vi "ELVIS III v1.0 Write DO Block Bank B DMA.vi"(8 "error in (no error)":errorcluster, 9 "DO FIFO Clock Divisor":u16, 10 "Bank Data":T1 caption="DO (N Samples) Configuration", 11 "FPGA Reference out":T3) -> (0 "error out":errorcluster)   [LabVIEW 2021]
uses:
  <vilib>/myRIO/Common/Instrument Driver Framework/Utilities/typedefs/Generic FPGA Reference.ctl
  <vilib>/myRIO/Common/Instrument Driver Framework/ELVIS III v1.0/DO Block/typedefs/ELVIS III DO Block Bank Data.ctl
  <vilib>/myRIO/Common/Instrument Driver Framework/ELVIS III v1.0/Resource Manager/typedefs/ELVIS III v1.0 Connector List.ctl
  <vilib>/myRIO/Common/Instrument Driver Framework/ELVIS III v1.0/DO Block/typedefs/ELVIS III DO Block FPGA Reference.ctl
  <vilib>/Utility/error.llb/Error Cluster From Error Code.vi
  <vilib>/rvi/errors/niLvFpgaAdjustHostInterfaceError.vi
  <vilib>/rvi/interface/nirviReadWriteControl/nirviReadWriteControl.xnode
  <vilib>/rvi/interface/nirviMethod/nirviMethod.xnode
  NiFpgaLv.dll
  <vilib>/rvi/interface/Simulation/niFpgaSimulationCallBeginRW.vi
  <vilib>/FPGAPlugInAG/Dynamic/niLvFpga_WriteFifo_Dynamic.vi
  <vilib>/rvi/errors/niLvFpgaMergeErrorWithErrorCode.vi
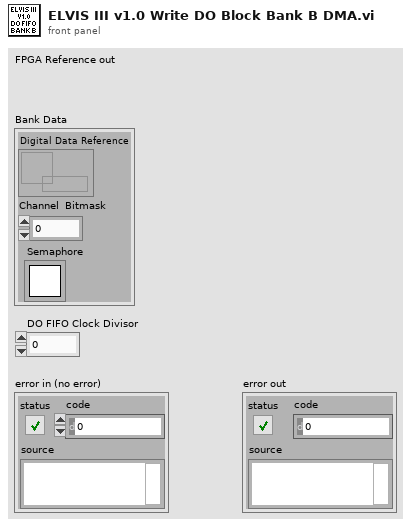
[diagram p1: front panel]
types:
  T1 = typedef "ELVIS III DO Block Bank Data.ctl" = cluster{"Digital Data Reference":refnum<data-value>, "Channel  Bitmask":fxp<+,20,20>, "Semaphore":T2}
  T2 = typedef "Semaphore RefNum" = refnum<k1>
  T3 = typedef "Generic FPGA Reference.ctl" = refnum<k20>
  T4 = typedef "ELVIS III v1.0 Connector List.ctl" = enum32{"None", "ConnectorA", "ConnectorB"}
  T5 = typedef "ELVIS III DO Block FPGA Reference.ctl" = refnum<k20>
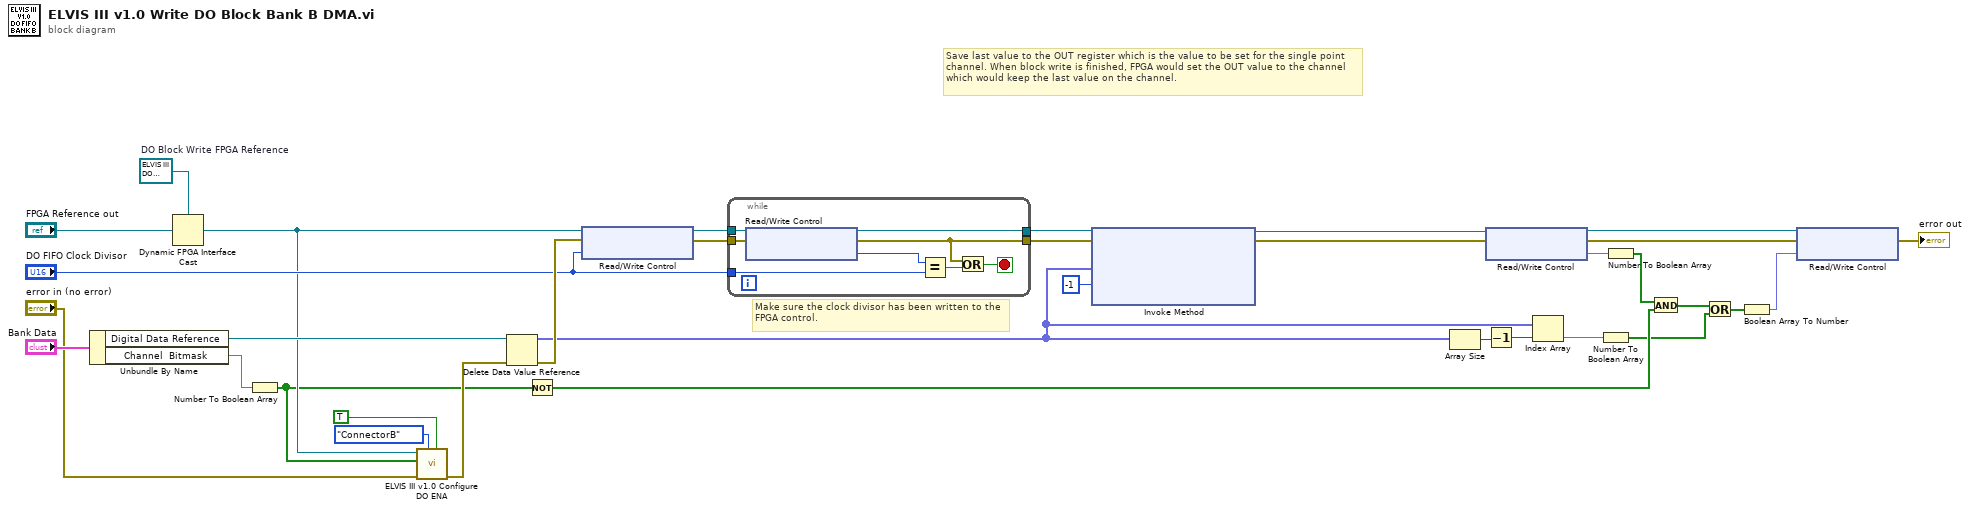
[diagram p0: block diagram]
diagram:
  w34 = T5 refnum  # DO Block Write FPGA Reference
  # "Save last value to the OUT register which is the value to be set for the single point channel. When block write is finished, FPGA would set the OUT value to the channel which would keep the last value on the channel."
  # "Make sure the clock divisor has been written to the FPGA control."
  n1 = Unbundle By Name("Bank Data") -> ("Digital Data Reference"=w14:refnum<data-value>, "Channel  Bitmask"=w13:fxp<+,20,20>)
  n2 = Dynamic FPGA Interface Cast(Session In=w34, Type="FPGA Reference out") -> (Session Out=w4:T5)
  n3 = Number To Boolean Array(number=w13) -> (Boolean array=w3:bool[])
  n4 = call <vilib>:"ELVIS III v1.0 Configure DO ENA.vi"("Apply Bitmask?"=TRUE, "Connector List"=ELVIS_III_v1.0_Connector_List."ConnectorB", "error in (no error)"="error in (no error)", "Bitmask Array"=w3, "myRIO FPGA Ref In"=w4) -> ("error out"=w5:errorcluster)  [unwired: 6 in]
  n5 = Delete Data Value Reference(data value reference=w14, error in=w5) -> (data value=w23:fxp<+,20,20>[], error out=w25:errorcluster)
  n6 = Not(x=w3) -> (.not. x?=w18:bool[])
  n7 = xnode "Read/Write Control"("FPGA VI Reference In"=w4, "error in"=w25, "DO.B.DMA_CNTR"="DO FIFO Clock Divisor") -> ("FPGA VI Reference Out"=w33:T5, "error out"=w32:errorcluster)
  n8 = while {
    tunnel: w33 -> [w42]
    tunnel: [w41] -> w27
    tunnel: [w37] -> w26
    tunnel: w32 -> [w40]
    tunnel: "DO FIFO Clock Divisor" -> [w39]
    stop <- w36 stop-if-true
    n9 = xnode "Read/Write Control"("FPGA VI Reference In"=w42, "error in"=w40) -> ("FPGA VI Reference Out"=w41:T5, "error out"=w37:errorcluster, "DO.B.DMA_CNTR"=w35:u16)
    n10 = Equal?(x=w35, y=w39) -> (x = y?=w38:bool)
    n11 = Or(x=w37, y=w38) -> (x .or. y?=w36:bool)
  }
  n12 = xnode "Invoke Method"("FPGA VI Reference In"=w27, "error in"=w26, "Data"=w23, "Timeout (ms)"=-1) -> ("FPGA VI Reference Out"=w2:T5, "error out"=w1:errorcluster)  [unwired: 1 out]
  n13 = Array Size(array=w23) -> (size(s)=w24:i32)
  n14 = xnode "Read/Write Control"("FPGA VI Reference In"=w2, "error in"=w1) -> ("FPGA VI Reference Out"=w29:T5, "error out"=w30:errorcluster, "DIO.B_19:0.OUT"=w22:fxp<+,20,20>)
  n15 = Decrement(x=w24) -> (x-1=w28:i32)
  n16 = Index Array(array=w23, index=w28) -> (element=w17:fxp<+,20,20>)
  n17 = Number To Boolean Array(number=w17) -> (Boolean array=w16:bool[])
  n18 = Number To Boolean Array(number=w22) -> (Boolean array=w19:bool[])
  n19 = And(x=w19, y=w18) -> (x .and. y?=w21:bool[])
  n20 = Or(x=w21, y=w16) -> (x .or. y?=w20:bool[])
  n21 = Boolean Array To Number(Boolean array=w20) -> (number=w15:fxp<+,20,20>)
  n22 = xnode "Read/Write Control"("FPGA VI Reference In"=w29, "error in"=w30, "DIO.B_19:0.OUT"=w15) -> ("error out"=→"error out":errorcluster)  [unwired: 1 out]
